vi "Update Numeric Value.vi"(7 "Init Refs":T3, 9 "Tree Data in":cluster{"Tag":string[], "Settings":T1[]} {"Settings"."Data Type" items=["Tree Parent"=-1, "Numeric"=0, "String"=1, "Boolean"=2, "Enum"=3]}, 10 "Settings In":T4, 11 "Tree Tag":string) -> (1 "Tree Data out":cluster{"Tag":string[], "Settings":T1[]} {"Settings"."Data Type" items=["Tree Parent"=-1, "Numeric"=0, "String"=1, "Boolean"=2, "Enum"=3]}, 2 "Settings In out":T4, 3 "New Tree Value":string)   [LabVIEW 2024, in "Sequencer with Output Values.lvlib" / "Sequencer with Output Values.lvclass"]
uses:
  Sequencer with Output Values.lvclass
  Params.ctl
  Step Settings.ctl
  Control Refs.ctl
  Tree Item Settings.ctl
  Data Type.ctl
  Global Tree Data.vi
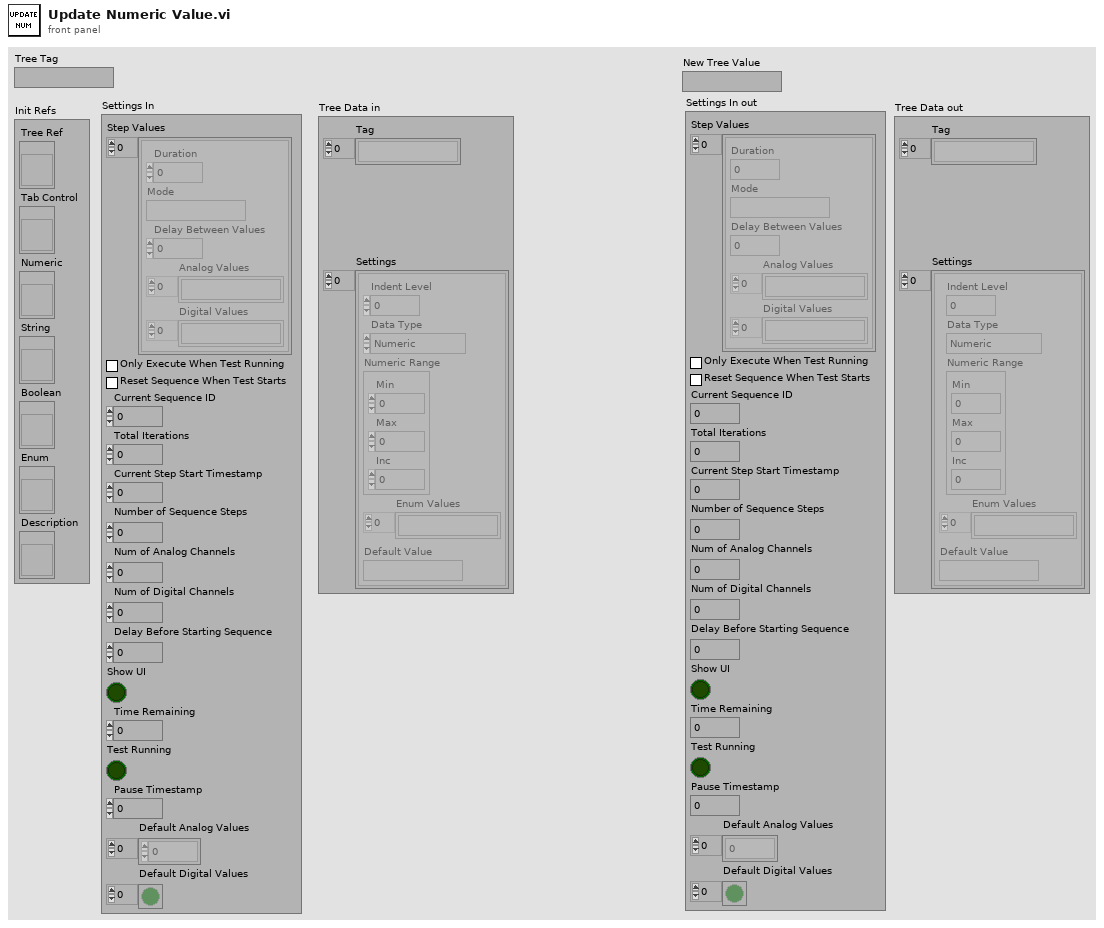
[diagram p1: front panel]
types:
  T1 = typedef "Sequencer with Output Values.lvlib/Sequencer with Output Values.lvclass/Tree Item Settings.ctl" = cluster{"Indent Level":i32, "Data Type":T2, "Numeric Range":cluster{"Min":dbl, "Max":dbl, "Inc":dbl}, "Enum Values":string[], "Default Value":string}
  T2 = typedef "Sequencer with Output Values.lvlib/Sequencer with Output Values.lvclass/Data Type.ctl" = i16
  T3 = typedef "Sequencer with Output Values.lvlib/Sequencer with Output Values.lvclass/Control Refs.ctl" = cluster{"Tree Ref":refnum<vi>, "Tab Control":refnum<vi>, "Numeric":refnum<vi>, "String":refnum<vi>, "Boolean":refnum<vi>, "Enum":refnum<vi>, "Description":refnum<vi>}
  T4 = typedef "Sequencer with Output Values.lvlib/Sequencer with Output Values.lvclass/Params.ctl" = cluster{"Step Values":T5[], "Only Execute When Test Running":bool, "Reset Sequence When Test Starts":bool, "Current Sequence ID":u32, "Total Iterations":u32, "Current Step Start Timestamp":dbl, "Number of Sequence Steps":i32, "Num of Analog Channels":i32, "Num of Digital Channels":i32, "Delay Before Starting Sequence":dbl, "Show UI":bool, "Time Remaining":dbl, "Test Running":bool, "Pause Timestamp":dbl, "Default Analog Values":dbl[], "Default Digital Values":bool[]}
  T5 = typedef "Sequencer with Output Values.lvlib/Sequencer with Output Values.lvclass/Step Settings.ctl" = cluster{"Duration":dbl, "Mode":string, "Delay Between Values":dbl, "Analog Values":string[], "Digital Values":string[]}
  T6 = cluster{"Left Cell String":string, "Child Text":string[], "Child Tag":string, "Item Indent":i32, "Child Only?":bool, "Glyph Index":i32}[]
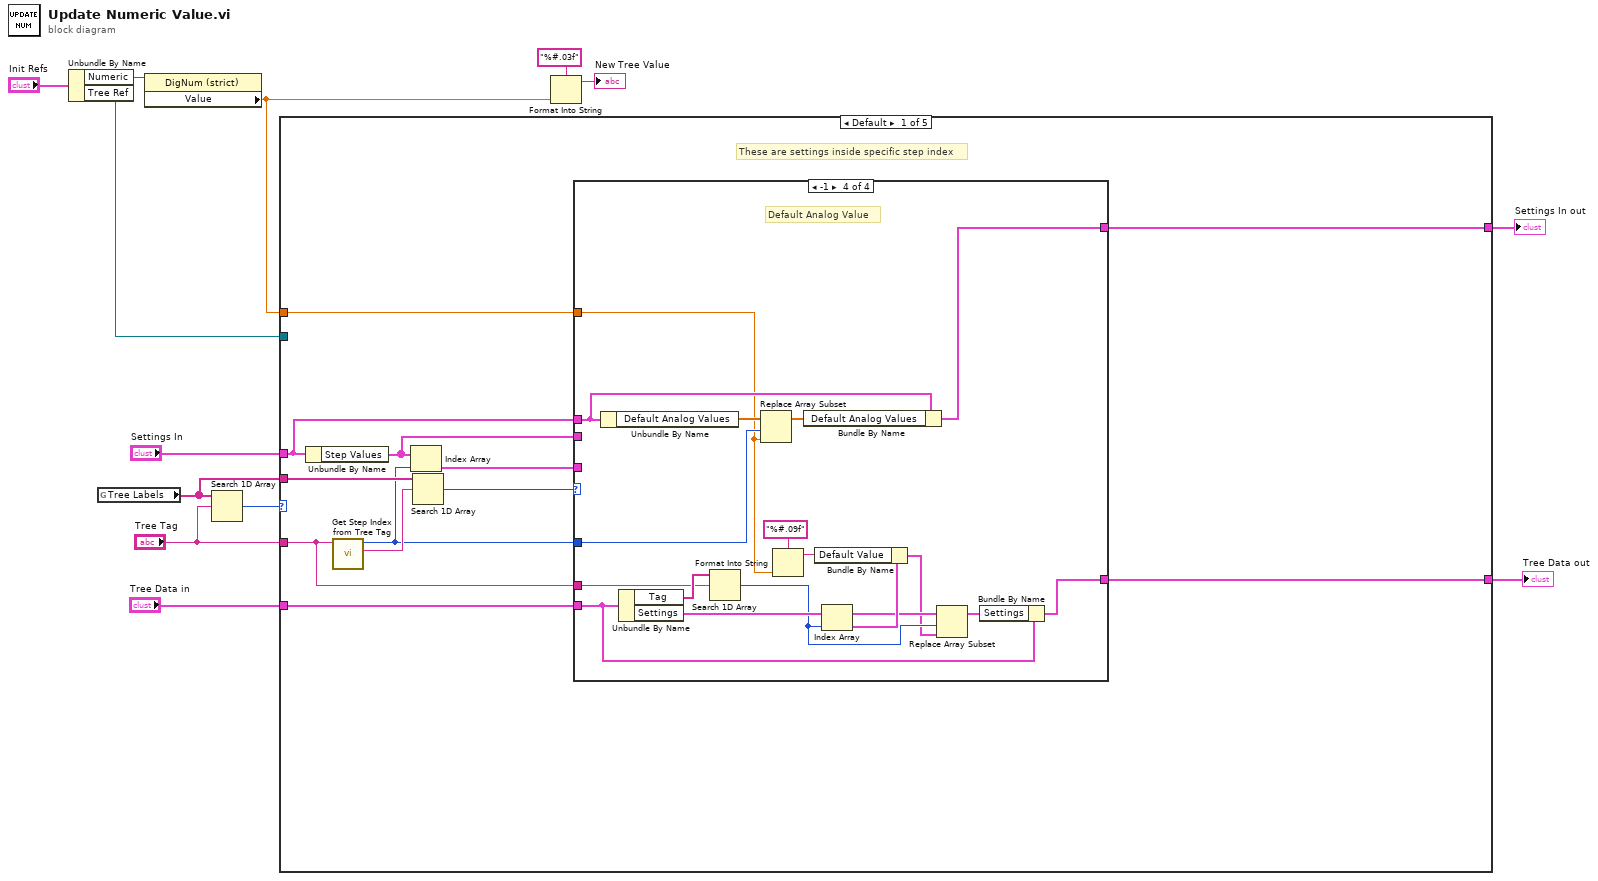
[diagram p0: block diagram]
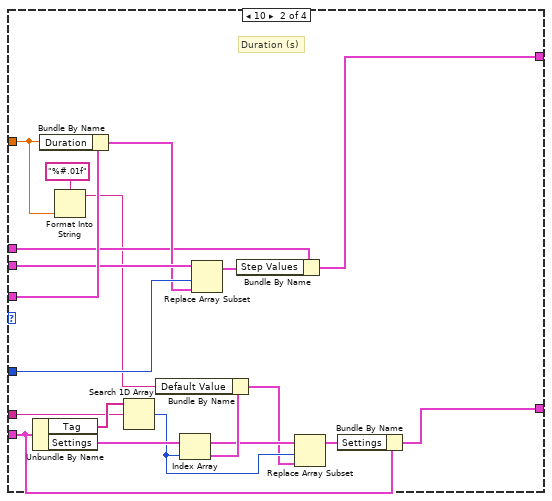
[diagram p3: hidden frame]
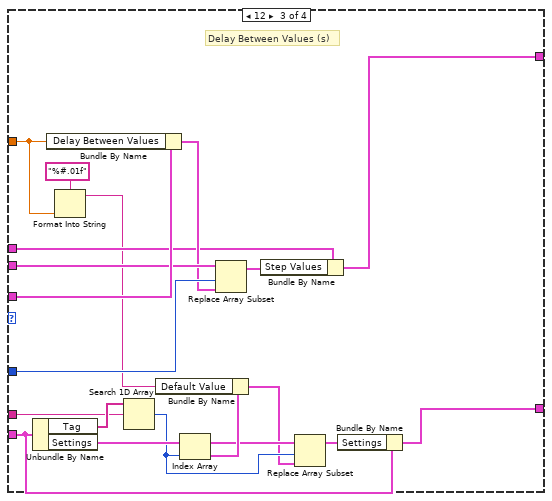
[diagram p4: hidden frame]
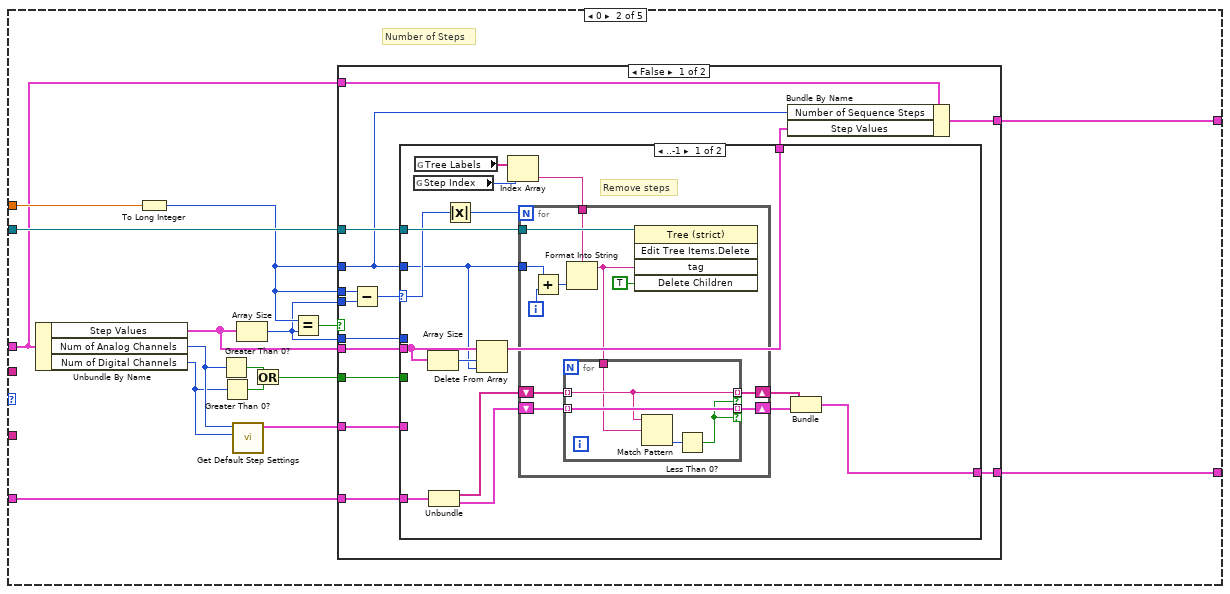
[diagram p5: hidden frame]
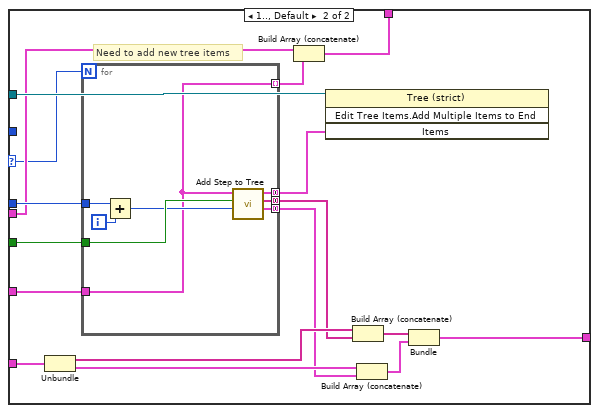
[diagram p6: hidden frame]
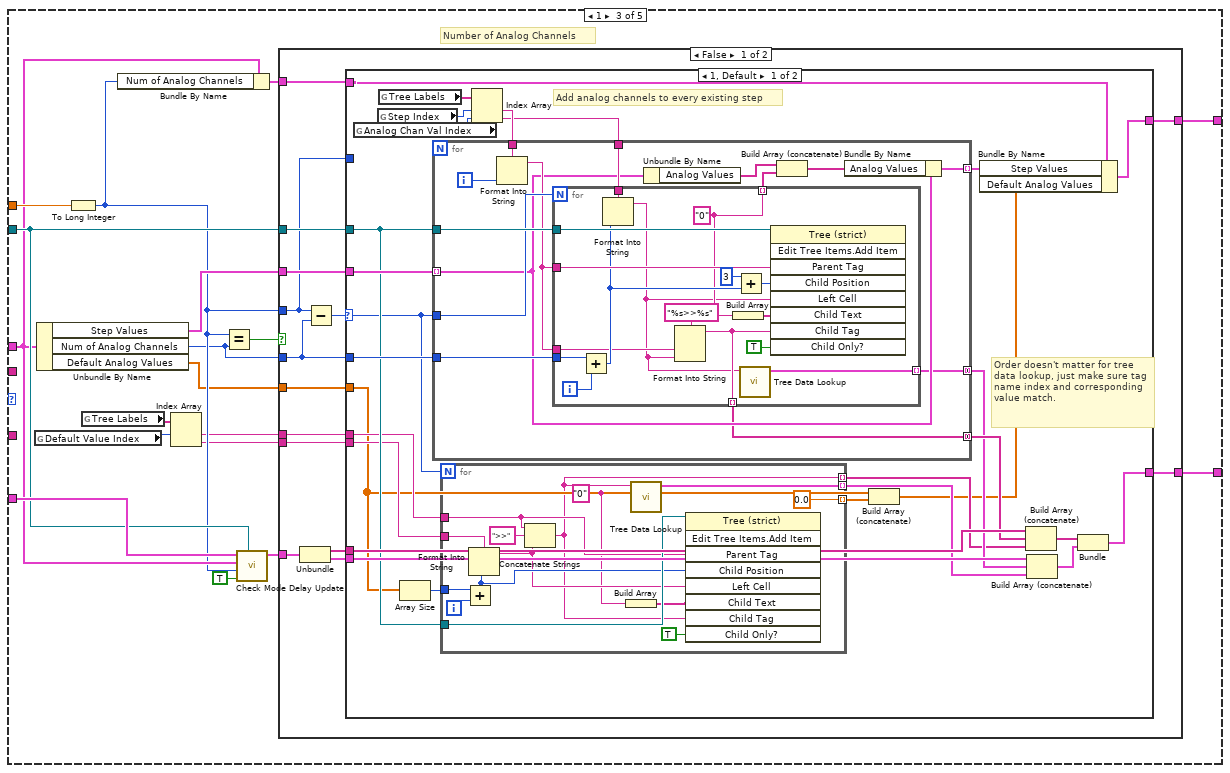
[diagram p8: hidden frame]
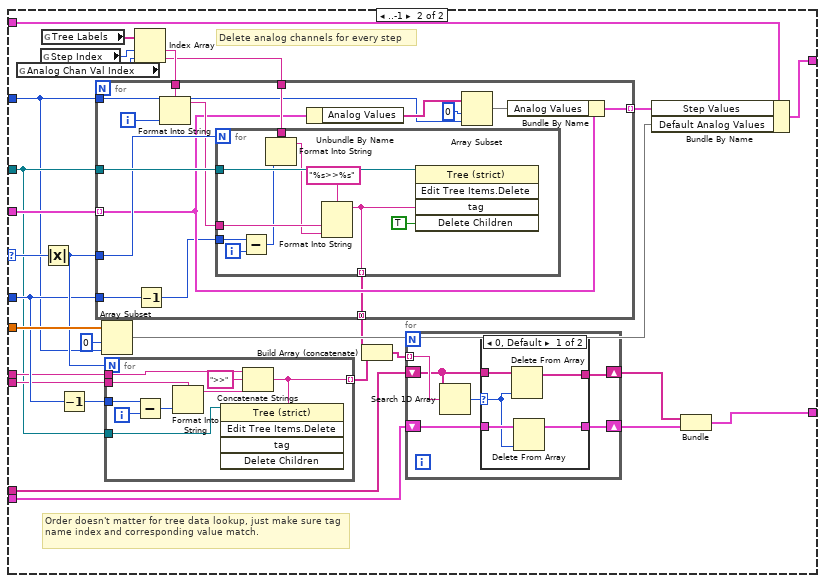
[diagram p9: hidden frame]
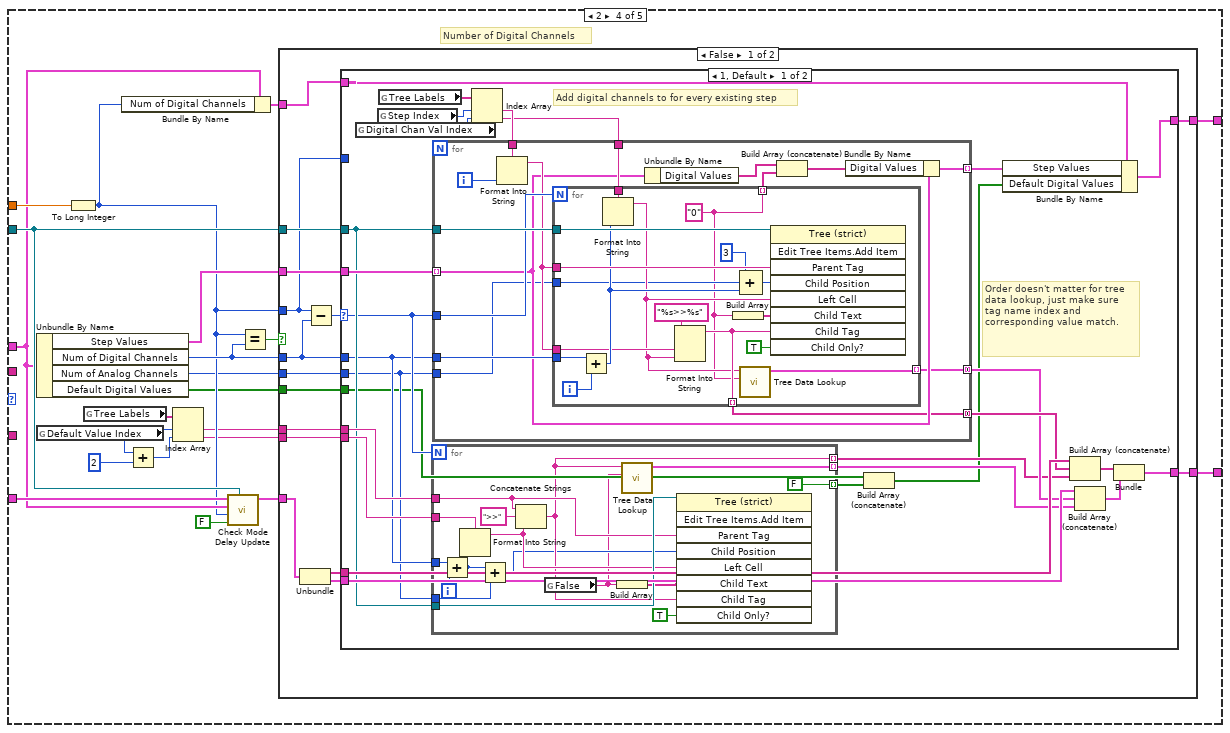
[diagram p12: hidden frame]
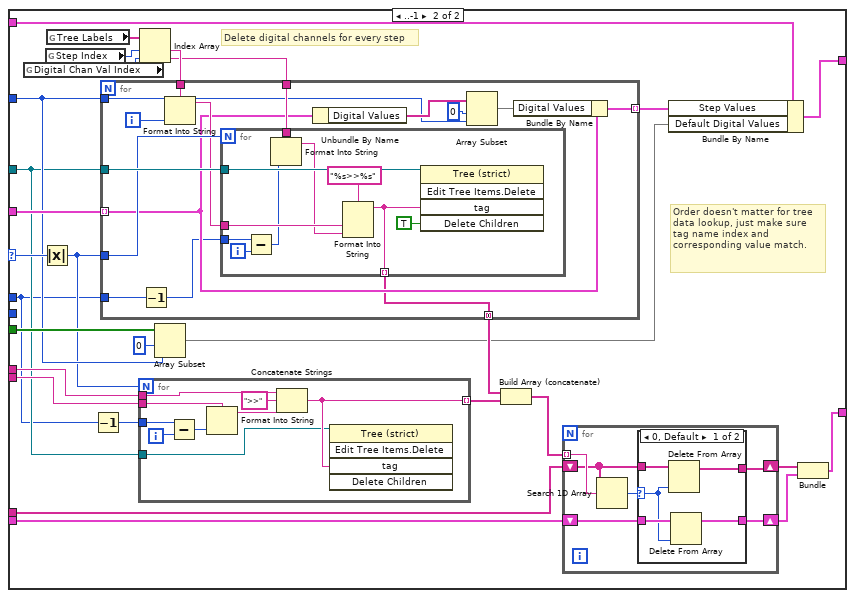
[diagram p13: hidden frame]
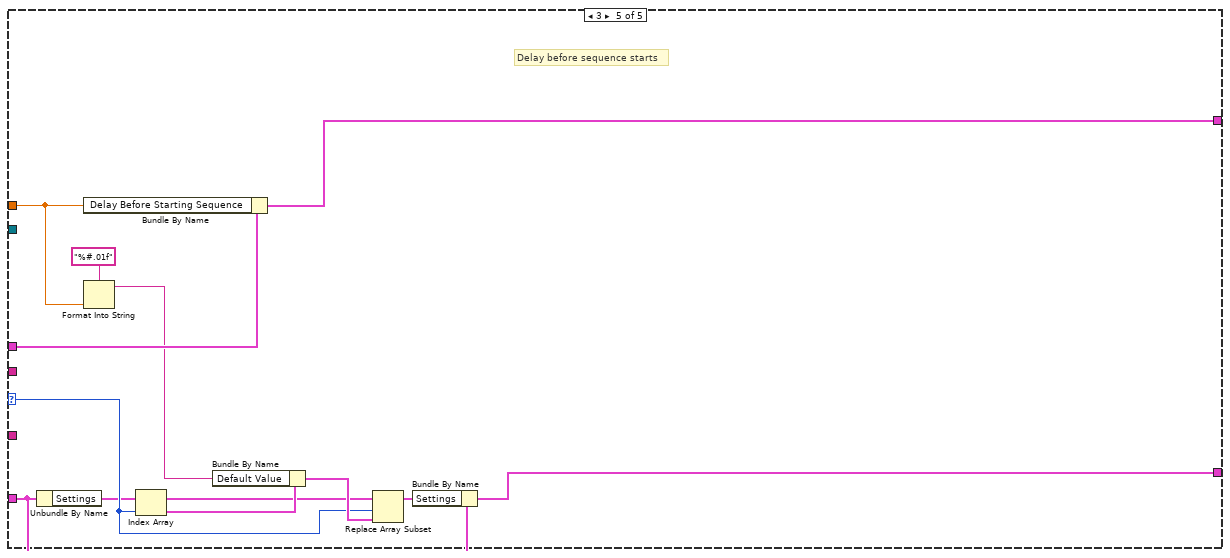
[diagram p16: hidden frame]
diagram:
  n1 = Unbundle By Name("Init Refs") -> ("Numeric"=w11:refnum<vi>, "Tree Ref"=w3:refnum<vi>)
  n2 = global read "Global Tree Data.vi" "Tree Labels"() -> (w1:string[])
  n3 = property class="DigNum (strict)"(reference=w11) -> ("Value"=w8:dbl)  [unwired: 1 in, 2 out]
  n4 = Search 1D Array(1D array=w1, element="Tree Tag") -> (index of element=w9:i32)  [unwired: 1 in]
  n5 = case shown="Default" w9 {
    selector: w9 -> [_ _ _ _ w544]
    tunnel: w8 -> [w21 w98 w189 w372 w548]
    tunnel: w3 -> [_ w96 w182 w363 _]
    tunnel: "Settings In" -> [w19 w87 w180 w362 w551]
    tunnel: "Tree Data in" -> [w20 w89 w183 w365 w543]
    tunnel: [w14 w88 w186 w369 w540] -> w5
    tunnel: [w16 w83 w187 w370 w550] -> w4
    tunnel: "Tree Tag" -> [w15 _ _ _ _]
    tunnel: w1 -> [w25 _ _ _ _]
    frame Default {
      # "These are settings inside specific step index"
      n6 = Unbundle By Name(w19) -> ("Step Values"=w18:T5[])
      n7 = call "Get Step Index from Tree Tag.vi"("Tree Tag"=w15) -> ("Step Param String"=w24:string, "Step Index"=w17:i32)  [unwired: 9 in]
      n8 = Index Array(array=w18, index=w17) -> (element=w23:T5)
      n9 = Search 1D Array(1D array=w25, element=w24) -> (index of element=w22:i32)  [unwired: 1 in]
      n10 = case shown="-1" w22 {
        tunnel: w23 -> [_ w46 w65 _]
        tunnel: w21 -> [_ w36 w55 w68]
        tunnel: w20 -> [w26 w30 w49 w69]
        tunnel: w19 -> [w27 w42 w61 w80]
        tunnel: w18 -> [_ w45 w64 _]
        tunnel: w17 -> [_ w44 w63 w81]
        tunnel: [w27 w40 w59 w78] -> w16
        tunnel: w15 -> [_ w38 w57 w71]
        tunnel: [w26 w28 w47 w70] -> w14
        frame Default {
        }
        frame 10 {
          # "Duration (s)"
          n11 = Unbundle By Name(w30) -> ("Tag"=w39:string[], "Settings"=w33:T1[])
          n12 = Bundle By Name(cluster=w46, "Duration"=w36) -> (w43:T5)
          n13 = Format Into String(format string="%#.01f", w36) -> (resulting string=w34:string)  [unwired: 2 in, 1 out]
          n14 = Search 1D Array(1D array=w39, element=w38) -> (index of element=w32:i32)  [unwired: 1 in]
          n15 = Index Array(array=w33, index=w32) -> (element=w37:T1)
          n16 = Bundle By Name(cluster=w37, "Default Value"=w34) -> (w31:T1)
          n17 = Replace Array Subset(array=w45, new element=w43, index=w44) -> (w41:T5[])
          n18 = Bundle By Name(cluster=w42, "Step Values"=w41) -> (w40:T4)
          n19 = Replace Array Subset(array=w33, new element=w31, index=w32) -> (w29:T1[])
          n20 = Bundle By Name(cluster=w30, "Settings"=w29) -> (w28:cluster{"Tag":string[], "Settings":T1[]})
        }
        frame 12 {
          # "Delay Between Values (s)"
          n21 = Unbundle By Name(w49) -> ("Tag"=w58:string[], "Settings"=w52:T1[])
          n22 = Bundle By Name(cluster=w65, "Delay Between Values"=w55) -> (w62:T5)
          n23 = Format Into String(format string="%#.01f", w55) -> (resulting string=w53:string)  [unwired: 2 in, 1 out]
          n24 = Search 1D Array(1D array=w58, element=w57) -> (index of element=w51:i32)  [unwired: 1 in]
          n25 = Index Array(array=w52, index=w51) -> (element=w56:T1)
          n26 = Bundle By Name(cluster=w56, "Default Value"=w53) -> (w50:T1)
          n27 = Replace Array Subset(array=w64, new element=w62, index=w63) -> (w60:T5[])
          n28 = Bundle By Name(cluster=w61, "Step Values"=w60) -> (w59:T4)
          n29 = Replace Array Subset(array=w52, new element=w50, index=w51) -> (w48:T1[])
          n30 = Bundle By Name(cluster=w49, "Settings"=w48) -> (w47:cluster{"Tag":string[], "Settings":T1[]})
        }
        frame -1 {
          # "Default Analog Value"
          n31 = Unbundle By Name(w80) -> ("Default Analog Values"=w82:dbl[])
          n32 = Unbundle By Name(w69) -> ("Tag"=w77:string[], "Settings"=w75:T1[])
          n33 = Search 1D Array(1D array=w77, element=w71) -> (index of element=w74:i32)  [unwired: 1 in]
          n34 = Replace Array Subset(array=w82, new element=w68, index=w81) -> (w79:dbl[])
          n35 = Format Into String(format string="%#.09f", w68) -> (resulting string=w66:string)  [unwired: 2 in, 1 out]
          n36 = Bundle By Name(cluster=w80, "Default Analog Values"=w79) -> (w78:T4)
          n37 = Index Array(array=w75, index=w74) -> (element=w76:T1)
          n38 = Bundle By Name(cluster=w76, "Default Value"=w66) -> (w73:T1)
          n39 = Replace Array Subset(array=w75, new element=w73, index=w74) -> (w72:T1[])
          n40 = Bundle By Name(cluster=w69, "Settings"=w72) -> (w70:cluster{"Tag":string[], "Settings":T1[]})
        }
      }
    }
    frame 0 {
      # "Number of Steps"
      n41 = Unbundle By Name(w87) -> ("Step Values"=w95:T5[], "Num of Analog Channels"=w86:i32, "Num of Digital Channels"=w85:i32)
      n42 = To Long Integer(number=w98) -> (32bit integer=w94:i32)
      n43 = Greater Than 0?(x=w86) -> (x > 0?=w92:bool)
      n44 = Greater Than 0?(x=w85) -> (x > 0?=w91:bool)
      n45 = call "Get Default Step Settings.vi"("Num of Digital Channels"=w85, "Num of Analog Channels"=w86) -> ("Default Step Settings"=w84:T5)  [unwired: 9 in]
      n46 = Array Size(array=w95) -> (size(s)=w93:i32)
      n47 = Or(x=w92, y=w91) -> (x .or. y?=w90:bool)
      n48 = Equal?(x=w94, y=w93) -> (x = y?=w97:bool)
      n49 = case shown="False" w97 {
        tunnel: w93 -> [w111 _]
        tunnel: w94 -> [w112 _]
        tunnel: w96 -> [w109 _]
        tunnel: w95 -> [w108 _]
        tunnel: w94 -> [w102 _]
        tunnel: w93 -> [w107 _]
        tunnel: w90 -> [w106 _]
        tunnel: w89 -> [w105 w170]
        tunnel: [w104 w170] -> w88
        tunnel: w87 -> [w103 w171]
        tunnel: w84 -> [w101 _]
        tunnel: [w99 w171] -> w83
        frame False {
          n50 = Subtract(x=w112, y=w111) -> (x-y=w110:i32)
          n51 = case shown="..-1" w110 {
            selector: w110 -> [w124 w145]
            tunnel: w109 -> [w125 w159]
            tunnel: w108 -> [w127 w146]
            tunnel: w102 -> [w121 _]
            tunnel: w107 -> [_ w161]
            tunnel: w106 -> [_ w160]
            tunnel: w105 -> [w122 w157]
            tunnel: [w113 w150] -> w104
            tunnel: w101 -> [_ w149]
            tunnel: [w128 w147] -> w100
            frame ..-1 {
              # "Remove steps"
              n52 = global read "Global Tree Data.vi" "Step Index"() -> (w119:i32)
              n53 = global read "Global Tree Data.vi" "Tree Labels"() -> (w120:string[])
              n54 = Array Size(array=w127) -> (size(s)=w126:i32)
              n55 = Unbundle(w122) -> ("Tag"=w117:string[], "Settings"=w116:T1[])
              n56 = Absolute Value(x=w124) -> (abs(x)=w123:i32)
              n57 = Delete From Array(array=w127, length=w126, index=w121) -> (array with subset deleted=w128:T5[])  [unwired: 1 out]
              n58 = Index Array(array=w120, index=w119) -> (element=w118:string)
              n59 = for {
                N: w123 -> [_]
                tunnel: w125 -> [w139]
                tunnel: w121 -> [w137]
                tunnel: w118 -> [w134]
                shift-right: [w131] -> w115
                shift-left: w117 -> [w133]
                shift-right: [w130] -> w114
                shift-left: w116 -> [w132]
                i -> [w136]
                n60 = Add(x=w137, y=w136) -> (x+y=w135:i32)
                n61 = Format Into String(format string=w134, w135) -> (resulting string=w129:string)  [unwired: 2 in, 1 out]
                n62 = for {
                  tunnel: w133 -> [w143] mode=indexing
                  tunnel: w132 -> [w144] mode=indexing
                  tunnel: [w143] -> w131 mode=indexing if=w140
                  tunnel: [w144] -> w130 mode=indexing if=w140
                  tunnel: w129 -> [w142]
                  n63 = Match Pattern(string=w143, regular expression=w142) -> (offset past match=w141:i32)  [unwired: 1 in, 3 out]
                  n64 = Less Than 0?(x=w141) -> (x < 0?=w140:bool)
                }
                n65 = invoke class="Tree (strict)" method="Edit Tree Items.Delete"(reference=w139, "tag"=w129, "Delete Children"=TRUE ("Delete Children?")) -> ()  [unwired: 2 in, 5 out]
              }
              n66 = Bundle("Tag"=w115, "Settings"=w114) -> (w113:cluster{"Tag":string[], "Settings":T1[]})  [unwired: 1 in]
            }
            frame 1.., Default {
              # "Need to add new tree items"
              n67 = Unbundle(w157) -> ("Tag"=w156:string[], "Settings"=w154:T1[])
              n68 = for {
                N: w145 -> [_]
                tunnel: w161 -> [w169]
                tunnel: w160 -> [w167]
                tunnel: [w165] -> w158 mode=concatenating
                tunnel: [w164] -> w155 mode=concatenating
                tunnel: [w163] -> w153 mode=concatenating
                tunnel: w149 -> [w162]
                tunnel: [w162] -> w148 mode=indexing
                i -> [w168]
                n69 = Add(x=w169, y=w168) -> (x+y=w166:i32)
                n70 = call "Add Step to Tree.vi"("Step Index"=w166, "Channels Defined"=w167, "Step Settings"=w162) -> ("Tree Data"=w163:T1[], "Tree Tags"=w164:string[], "Tree Items"=w165:T6)  [unwired: 6 in]
              }
              n71 = Build Array (concatenate)(w146, w148) -> (w147:T5[])
              n72 = invoke class="Tree (strict)" method="Edit Tree Items.Add Multiple Items to End"(reference=w159, "Items"=w158) -> ()  [unwired: 2 in, 4 out]
              n73 = Build Array (concatenate)(w156, w155) -> (w152:string[])
              n74 = Build Array (concatenate)(w154, w153) -> (w151:T1[])
              n75 = Bundle(w152, w151) -> (w150:cluster{string[], T1[]})  [unwired: 1 in]
            }
          }
          n76 = Bundle By Name(cluster=w103, "Number of Sequence Steps"=w102, "Step Values"=w100) -> (w99:T4)
        }
        frame True {
          # "Didn't change, so nothing to do."
        }
      }
    }
    frame 1 {
      # "Number of Analog Channels"
      n77 = global read "Global Tree Data.vi" "Default Value Index"() -> (w174:i32)
      n78 = Unbundle By Name(w180) -> ("Step Values"=w185:T5[], "Num of Analog Channels"=w177:i32, "Default Analog Values"=w176:dbl[])
      n79 = To Long Integer(number=w189) -> (32bit integer=w179:i32)
      n80 = global read "Global Tree Data.vi" "Tree Labels"() -> (w175:string[])
      n81 = Bundle By Name(cluster=w180, "Num of Analog Channels"=w179) -> (w178:T4)
      n82 = Index Array(array=w175, index #1=w174) -> (element #1=w172:string, element #2=w173:string)  [unwired: 1 in]
      n83 = Equal?(x=w179, y=w177) -> (x = y?=w188:bool)
      n84 = call "Check Mode Delay Update.vi"("TreeControl in"=w182, "Analog Changed"=TRUE, "New Num"=w179, "Settings In in"=w180, "Tree Data in"=w183) -> ("Tree Data out"=w184:cluster{"Tag":string[], "Settings":T1[]})  [unwired: 6 in]
      n85 = case shown="False" w188 {
        tunnel: w178 -> [w199 w351]
        tunnel: [w198 w351] -> w187
        tunnel: w184 -> [w197 w350]
        tunnel: [w194 w350] -> w186
        tunnel: w177 -> [w200 _]
        tunnel: w179 -> [w193 _]
        tunnel: w182 -> [w202 _]
        tunnel: w185 -> [w201 _]
        tunnel: w176 -> [w192 _]
        tunnel: w173 -> [w191 _]
        tunnel: w172 -> [w190 _]
        frame False {
          n86 = Unbundle(w197) -> ("Tag"=w196:string[], "Settings"=w195:T1[])
          n87 = Subtract(x=w193, y=w200) -> (x-y=w203:i32)
          n88 = case shown="1, Default" w203 {
            selector: w203 -> [w208 w298]
            tunnel: w202 -> [w211 w276]
            tunnel: w201 -> [w230 w302]
            tunnel: w200 -> [w226 w281]
            tunnel: w199 -> [w223 w295]
            tunnel: [w221 w293] -> w198
            tunnel: w196 -> [w220 w291]
            tunnel: w195 -> [w218 w290]
            tunnel: [w214 w292] -> w194
            tunnel: w193 -> [_ w275]
            tunnel: w192 -> [w205 w287]
            tunnel: w191 -> [w209 w279]
            tunnel: w190 -> [w210 w277]
            frame 1, Default {
              # "Order doesn't matter for tree data lookup, just make sure tag name index and corresponding value match."
              # "Add analog channels to every existing step"
              n89 = global read "Global Tree Data.vi" "Analog Chan Val Index"() -> (w225:i32)
              n90 = global read "Global Tree Data.vi" "Step Index"() -> (w229:i32)
              n91 = global read "Global Tree Data.vi" "Tree Labels"() -> (w228:string[])
              n92 = Array Size(array=w205) -> (size(s)=w207:i32)
              n93 = for {
                N: w208 -> [_]
                tunnel: [w243] -> w212 mode=indexing
                tunnel: [w233] -> w213 mode=indexing
                tunnel: w211 -> [w242]
                tunnel: w210 -> [w238]
                tunnel: w209 -> [w241]
                tunnel: w207 -> [w239]
                tunnel: [0.0] -> w206 mode=indexing
                i -> [w240]
                w235 = "0" ("Value")
                n94 = Add(x=w239, y=w240) -> (x+y=w237:i32)
                n95 = Format Into String(format string=w241, w237) -> (resulting string=w236:string)  [unwired: 2 in, 1 out]
                n96 = Concatenate Strings(w238, ">>" ("string"), w236) -> (w233:string)
                n97 = Build Array(w235) -> (w234:string[])
                n98 = call "Tree Data Lookup.vi"("Value"=w235, "Key"=w233) -> ("Tree Data"=w243:T1)  [unwired: 9 in]
                n99 = invoke class="Tree (strict)" method="Edit Tree Items.Add Item"(reference=w242, "Parent Tag"=w238, "Child Position"=w237, "Left Cell"=w236, "Child Text"=w234, "Child Tag"=w233, "Child Only?"=TRUE) -> ()  [unwired: 2 in, 9 out]
              }
              n100 = Index Array(array=w228, index #1=w229, index #2=w225) -> (element #1=w227:string, element #2=w224:string)
              n101 = for {
                tunnel: w211 -> [w258]
                tunnel: w230 -> [w251] mode=indexing
                tunnel: w227 -> [w257]
                tunnel: w226 -> [w255]
                tunnel: w208 -> [w254]
                tunnel: w224 -> [w253]
                tunnel: [w247] -> w222 mode=indexing
                tunnel: [w246] -> w219 mode=concatenating
                tunnel: [w245] -> w217 mode=concatenating
                i -> [w256]
                n102 = Format Into String(format string=w257, w256) -> (resulting string=w252:string)  [unwired: 2 in, 1 out]
                n103 = for {
                  N: w254 -> [_]
                  tunnel: w258 -> [w274]
                  tunnel: w255 -> [w273]
                  tunnel: w253 -> [w271]
                  tunnel: w252 -> [w270]
                  tunnel: w252 -> [w265]
                  tunnel: [w263] -> w249 mode=indexing
                  tunnel: [w262] -> w246 mode=indexing
                  tunnel: [w260] -> w245 mode=indexing
                  i -> [w272]
                  w263 = "0"
                  n104 = Add(x=w273, y=w272) -> (x+y=w268:i32)
                  n105 = Format Into String(format string=w271, w268) -> (resulting string=w261:string)  [unwired: 2 in, 1 out]
                  n106 = Format Into String(format string="%s>>%s" ("string"), w265, w261) -> (resulting string=w262:string)  [unwired: 2 in, 1 out]
                  n107 = Build Array(w263) -> (w259:string[])
                  n108 = Add(x=3, y=w268) -> (x+y=w267:i32)
                  n109 = call "Tree Data Lookup.vi"("Key"=w261) -> ("Tree Data"=w260:T1)  [unwired: 10 in]
                  n110 = invoke class="Tree (strict)" method="Edit Tree Items.Add Item"(reference=w274, "Parent Tag"=w270, "Child Position"=w267, "Left Cell"=w261, "Child Text"=w259, "Child Tag"=w262, "Child Only?"=TRUE) -> ()  [unwired: 2 in, 9 out]
                }
                n111 = Unbundle By Name(w251) -> ("Analog Values"=w250:string[])
                n112 = Build Array (concatenate)(w250, w249) -> (w248:string[])
                n113 = Bundle By Name(cluster=w251, "Analog Values"=w248) -> (w247:T5)
              }
              n114 = Build Array (concatenate)(w205, w206) -> (w204:dbl[])
              n115 = Bundle By Name(cluster=w223, "Step Values"=w222, "Default Analog Values"=w204) -> (w221:T4)
              n116 = Build Array (concatenate)(w220, w219, w213) -> (w216:string[])
              n117 = Build Array (concatenate)(w218, w217, w212) -> (w215:T1[])
              n118 = Bundle(w216, w215) -> (w214:cluster{string[], T1[]})  [unwired: 1 in]
            }
            frame ..-1 {
              # "Order doesn't matter for tree data lookup, just make sure tag name index and corresponding value match."
              # "Delete analog channels for every step"
              n119 = global read "Global Tree Data.vi" "Analog Chan Val Index"() -> (w297:i32)
              n120 = global read "Global Tree Data.vi" "Step Index"() -> (w301:i32)
              n121 = global read "Global Tree Data.vi" "Tree Labels"() -> (w300:string[])
              n122 = Absolute Value(x=w298) -> (abs(x)=w284:i32)
              n123 = Decrement(x=w281) -> (x-1=w280:i32)
              n124 = Array Subset(array=w287, index=0, length=w275) -> (w285:dbl[])
              n125 = for {
                N: w284 -> [_]
                tunnel: w280 -> [w311]
                tunnel: w279 -> [w308]
                tunnel: w277 -> [w306]
                tunnel: [w304] -> w278 mode=indexing
                tunnel: w276 -> [w303]
                i -> [w310]
                n126 = Subtract(x=w311, y=w310) -> (x-y=w309:i32)
                n127 = Format Into String(format string=w308, w309) -> (resulting string=w305:string)  [unwired: 2 in, 1 out]
                n128 = Concatenate Strings(w306, ">>" ("string"), w305) -> (w304:string)
                n129 = invoke class="Tree (strict)" method="Edit Tree Items.Delete"(reference=w303, "tag"=w304) -> ()  [unwired: 3 in, 5 out]
              }
              n130 = Index Array(array=w300, index #1=w301, index #2=w297) -> (element #1=w299:string, element #2=w296:string)
              n131 = for {
                tunnel: w276 -> [w339]
                tunnel: w302 -> [w332] mode=indexing
                tunnel: w299 -> [w338]
                tunnel: w281 -> [w336]
                tunnel: w284 -> [w335]
                tunnel: w296 -> [w334]
                tunnel: [w331] -> w294 mode=indexing
                tunnel: [w330] -> w283 mode=concatenating
                tunnel: w275 -> [w326]
                i -> [w337]
                n132 = Decrement(x=w336) -> (x-1=w329:i32)
                n133 = Format Into String(format string=w338, w337) -> (resulting string=w333:string)  [unwired: 2 in, 1 out]
                n134 = for {
                  N: w335 -> [_]
                  tunnel: w339 -> [w349]
                  tunnel: w329 -> [w345]
                  tunnel: w334 -> [w348]
                  tunnel: w333 -> [w347]
                  tunnel: [w341] -> w330 mode=indexing
                  i -> [w344]
                  n135 = Subtract(x=w345, y=w344) -> (x-y=w343:i32)
                  n136 = Format Into String(format string=w348, w343) -> (resulting string=w346:string)  [unwired: 2 in, 1 out]
                  n137 = Format Into String(format string="%s>>%s", w347, w346) -> (resulting string=w341:string)  [unwired: 2 in, 1 out]
                  n138 = invoke class="Tree (strict)" method="Edit Tree Items.Delete"(reference=w349, "tag"=w341, "Delete Children"=TRUE ("Delete Children?")) -> ()  [unwired: 2 in, 5 out]
                }
                n139 = Unbundle By Name(w332) -> ("Analog Values"=w328:string[])
                n140 = Array Subset(array=w328, index=0, length=w326) -> (w327:string[])
                n141 = Bundle By Name(cluster=w332, "Analog Values"=w327) -> (w331:T5)
              }
              n142 = Build Array (concatenate)(w283, w278) -> (w282:string[])
              n143 = for {
                tunnel: w282 -> [w317] mode=indexing
                shift-right: [w314] -> w289
                shift-left: w291 -> [w315]
                shift-right: [w312] -> w288
                shift-left: w290 -> [w313]
                n144 = Search 1D Array(1D array=w315, element=w317) -> (index of element=w316:i32)  [unwired: 1 in]
                n145 = case shown="0, Default" w316 {
                  selector: w316 -> [w319 _]
                  tunnel: w315 -> [w322 w324]
                  tunnel: [w321 w324] -> w314
                  tunnel: w313 -> [w320 w323]
                  tunnel: [w318 w323] -> w312
                  frame 0, Default {
                    n146 = Delete From Array(array=w322, index=w319) -> (array with subset deleted=w321:string[])  [unwired: 1 in, 1 out]
                    n147 = Delete From Array(array=w320, index=w319) -> (array with subset deleted=w318:T1[])  [unwired: 1 in, 1 out]
                  }
                  frame -1 {
                  }
                }
              }
              n148 = Bundle By Name(cluster=w295, "Step Values"=w294, "Default Analog Values"=w285) -> (w293:T4)
              n149 = Bundle("Tag"=w289, "Settings"=w288) -> (w292:cluster{"Tag":string[], "Settings":T1[]})  [unwired: 1 in]
            }
          }
        }
        frame True {
        }
      }
    }
    frame 2 {
      # "Number of Digital Channels"
      n150 = Unbundle By Name(w362) -> ("Step Values"=w368:T5[], "Num of Digital Channels"=w367:i32, "Num of Analog Channels"=w359:i32, "Default Digital Values"=w352:bool[])
      n151 = global read "Global Tree Data.vi" "Default Value Index"() -> (w357:i32)
      n152 = To Long Integer(number=w372) -> (32bit integer=w361:i32)
      n153 = global read "Global Tree Data.vi" "Tree Labels"() -> (w358:string[])
      n154 = Bundle By Name(cluster=w362, "Num of Digital Channels"=w361) -> (w360:T4)
      n155 = Add(x=w357, y=2) -> (x+y=w355:i32)
      n156 = Index Array(array=w358, index #1=w357, index #2=w355) -> (element #1=w354:string, element #2=w353:string)
      n157 = call "Check Mode Delay Update.vi"("TreeControl in"=w363, "Analog Changed"=FALSE, "New Num"=w361, "Settings In in"=w362, "Tree Data in"=w365) -> ("Tree Data out"=w364:cluster{"Tag":string[], "Settings":T1[]})  [unwired: 6 in]
      n158 = Equal?(x=w361, y=w367) -> (x = y?=w371:bool)
      n159 = case shown="False" w371 {
        tunnel: w360 -> [w383 w539]
        tunnel: [w382 w539] -> w370
        tunnel: w364 -> [w381 w538]
        tunnel: [w378 w538] -> w369
        tunnel: w367 -> [w384 _]
        tunnel: w361 -> [w377 _]
        tunnel: w363 -> [w386 _]
        tunnel: w368 -> [w385 _]
        tunnel: w359 -> [w376 _]
        tunnel: w354 -> [w375 _]
        tunnel: w353 -> [w374 _]
        tunnel: w352 -> [w373 _]
        frame False {
          n160 = Unbundle(w381) -> ("Tag"=w380:string[], "Settings"=w379:T1[])
          n161 = Subtract(x=w377, y=w384) -> (x-y=w387:i32)
          n162 = case shown="1, Default" w387 {
            selector: w387 -> [w395 w486]
            tunnel: w386 -> [w396 w465]
            tunnel: w385 -> [w414 w490]
            tunnel: w384 -> [w394 w463]
            tunnel: w383 -> [w408 w483]
            tunnel: [w406 w481] -> w382
            tunnel: w380 -> [w405 w479]
            tunnel: w379 -> [w403 w478]
            tunnel: [w399 w480] -> w378
            tunnel: w377 -> [_ w470]
            tunnel: w376 -> [w393 _]
            tunnel: w375 -> [w398 w467]
            tunnel: w374 -> [w397 w466]
            tunnel: w373 -> [w389 w472]
            frame 1, Default {
              # "Order doesn't matter for tree data lookup, just make sure tag name index and corresponding value match."
              # "Add digital channels to for every existing step"
              n163 = global read "Global Tree Data.vi" "Digital Chan Val Index"() -> (w410:i32)
              n164 = global read "Global Tree Data.vi" "Step Index"() -> (w413:i32)
              n165 = global read "Global Tree Data.vi" "Tree Labels"() -> (w412:string[])
              n166 = for {
                N: w395 -> [_]
                tunnel: [w429] -> w391 mode=indexing
                tunnel: [w421] -> w392 mode=indexing
                tunnel: w396 -> [w428]
                tunnel: w398 -> [w424]
                tunnel: w397 -> [w427]
                tunnel: w394 -> [w425]
                tunnel: [FALSE] -> w390 mode=indexing
                tunnel: w393 -> [w417]
                i -> [w426]
                n167 = Add(x=w425, y=w426) -> (x+y=w418:i32)
                n168 = Format Into String(format string=w427, w418) -> (resulting string=w423:string)  [unwired: 2 in, 1 out]
                n169 = Add(x=w418, y=w417) -> (x+y=w416:i32)
                n170 = Concatenate Strings(w424, ">>" ("string"), w423) -> (w421:string)
                n171 = global read "Global Tree Data.vi" "False"() -> (w415:string)
                n172 = Build Array(w415) -> (w422:string[])
                n173 = call "Tree Data Lookup.vi"("Value"=w415, "Key"=w421) -> ("Tree Data"=w429:T1)  [unwired: 9 in]
                n174 = invoke class="Tree (strict)" method="Edit Tree Items.Add Item"(reference=w428, "Parent Tag"=w424, "Child Position"=w416, "Left Cell"=w423, "Child Text"=w422, "Child Tag"=w421, "Child Only?"=TRUE) -> ()  [unwired: 2 in, 9 out]
              }
              n175 = Index Array(array=w412, index #1=w413, index #2=w410) -> (element #1=w411:string, element #2=w409:string)
              n176 = for {
                tunnel: w396 -> [w445]
                tunnel: w414 -> [w438] mode=indexing
                tunnel: w411 -> [w444]
                tunnel: w394 -> [w442]
                tunnel: w395 -> [w441]
                tunnel: w409 -> [w440]
                tunnel: [w434] -> w407 mode=indexing
                tunnel: [w433] -> w404 mode=concatenating
                tunnel: [w432] -> w402 mode=concatenating
                tunnel: w393 -> [w431]
                i -> [w443]
                n177 = Format Into String(format string=w444, w443) -> (resulting string=w439:string)  [unwired: 2 in, 1 out]
                n178 = for {
                  N: w441 -> [_]
                  tunnel: w445 -> [w462]
                  tunnel: w442 -> [w461]
                  tunnel: w440 -> [w459]
                  tunnel: w439 -> [w458]
                  tunnel: w439 -> [w454]
                  tunnel: [w446] -> w436 mode=indexing
                  tunnel: [w452] -> w433 mode=indexing
                  tunnel: [w450] -> w432 mode=indexing
                  tunnel: w431 -> [w447]
                  i -> [w460]
                  w446 = "0"
                  n179 = Add(x=w461, y=w460) -> (x+y=w457:i32)
                  n180 = Format Into String(format string=w459, w457) -> (resulting string=w451:string)  [unwired: 2 in, 1 out]
                  n181 = Format Into String(format string="%s>>%s" ("string"), w454, w451) -> (resulting string=w452:string)  [unwired: 2 in, 1 out]
                  n182 = Build Array(w446) -> (w449:string[])
                  n183 = Compound Arithmetic op=ADD(3, w447, w457) -> (w456:i32)
                  n184 = call "Tree Data Lookup.vi"("Value"=w446, "Key"=w451) -> ("Tree Data"=w450:T1)  [unwired: 9 in]
                  n185 = invoke class="Tree (strict)" method="Edit Tree Items.Add Item"(reference=w462, "Parent Tag"=w458, "Child Position"=w456, "Left Cell"=w451, "Child Text"=w449, "Child Tag"=w452, "Child Only?"=TRUE) -> ()  [unwired: 2 in, 9 out]
                }
                n186 = Unbundle By Name(w438) -> ("Digital Values"=w437:string[])
                n187 = Build Array (concatenate)(w437, w436) -> (w435:string[])
                n188 = Bundle By Name(cluster=w438, "Digital Values"=w435) -> (w434:T5)
              }
              n189 = Build Array (concatenate)(w389, w390) -> (w388:bool[])
              n190 = Bundle By Name(cluster=w408, "Step Values"=w407, "Default Digital Values"=w388) -> (w406:T4)
              n191 = Build Array (concatenate)(w405, w404, w392) -> (w401:string[])
              n192 = Build Array (concatenate)(w403, w402, w391) -> (w400:T1[])
              n193 = Bundle(w401, w400) -> (w399:cluster{string[], T1[]})  [unwired: 1 in]
            }
            frame ..-1 {
              # "Order doesn't matter for tree data lookup, just make sure tag name index and corresponding value match."
              # "Delete digital channels for every step"
              n194 = global read "Global Tree Data.vi" "Digital Chan Val Index"() -> (w485:i32)
              n195 = Absolute Value(x=w486) -> (abs(x)=w469:i32)
              n196 = global read "Global Tree Data.vi" "Step Index"() -> (w489:i32)
              n197 = global read "Global Tree Data.vi" "Tree Labels"() -> (w488:string[])
              n198 = Decrement(x=w463) -> (x-1=w464:i32)
              n199 = for {
                N: w469 -> [_]
                tunnel: w464 -> [w499]
                tunnel: w466 -> [w496]
                tunnel: w467 -> [w494]
                tunnel: [w492] -> w473 mode=indexing
                tunnel: w465 -> [w491]
                i -> [w498]
                n200 = Subtract(x=w499, y=w498) -> (x-y=w497:i32)
                n201 = Format Into String(format string=w496, w497) -> (resulting string=w493:string)  [unwired: 2 in, 1 out]
                n202 = Concatenate Strings(w494, ">>" ("string"), w493) -> (w492:string)
                n203 = invoke class="Tree (strict)" method="Edit Tree Items.Delete"(reference=w491, "tag"=w492) -> ()  [unwired: 3 in, 5 out]
              }
              n204 = Index Array(array=w488, index #1=w489, index #2=w485) -> (element #1=w487:string, element #2=w484:string)
              n205 = for {
                tunnel: w465 -> [w527]
                tunnel: w490 -> [w520] mode=indexing
                tunnel: w487 -> [w526]
                tunnel: w463 -> [w524]
                tunnel: w469 -> [w523]
                tunnel: w484 -> [w522]
                tunnel: [w519] -> w482 mode=indexing
                tunnel: [w518] -> w475 mode=concatenating
                tunnel: w470 -> [w514]
                i -> [w525]
                n206 = Decrement(x=w524) -> (x-1=w517:i32)
                n207 = Format Into String(format string=w526, w525) -> (resulting string=w521:string)  [unwired: 2 in, 1 out]
                n208 = for {
                  N: w523 -> [_]
                  tunnel: w527 -> [w537]
                  tunnel: w517 -> [w533]
                  tunnel: w522 -> [w536]
                  tunnel: w521 -> [w535]
                  tunnel: [w529] -> w518 mode=indexing
                  i -> [w532]
                  n209 = Subtract(x=w533, y=w532) -> (x-y=w531:i32)
                  n210 = Format Into String(format string=w536, w531) -> (resulting string=w534:string)  [unwired: 2 in, 1 out]
                  n211 = Format Into String(format string="%s>>%s", w535, w534) -> (resulting string=w529:string)  [unwired: 2 in, 1 out]
                  n212 = invoke class="Tree (strict)" method="Edit Tree Items.Delete"(reference=w537, "tag"=w529, "Delete Children"=TRUE ("Delete Children?")) -> ()  [unwired: 2 in, 5 out]
                }
                n213 = Unbundle By Name(w520) -> ("Digital Values"=w516:string[])
                n214 = Array Subset(array=w516, index=0, length=w514) -> (w515:string[])
                n215 = Bundle By Name(cluster=w520, "Digital Values"=w515) -> (w519:T5)
              }
              n216 = Array Subset(array=w472, index=0, length=w470) -> (w468:bool[])
              n217 = Build Array (concatenate)(w475, w473) -> (w474:string[])
              n218 = for {
                tunnel: w474 -> [w505] mode=indexing
                shift-right: [w502] -> w477
                shift-left: w479 -> [w503]
                shift-right: [w500] -> w476
                shift-left: w478 -> [w501]
                n219 = Search 1D Array(1D array=w503, element=w505) -> (index of element=w504:i32)  [unwired: 1 in]
                n220 = case shown="0, Default" w504 {
                  selector: w504 -> [w507 _]
                  tunnel: w503 -> [w510 w512]
                  tunnel: [w509 w512] -> w502
                  tunnel: w501 -> [w508 w511]
                  tunnel: [w506 w511] -> w500
                  frame 0, Default {
                    n221 = Delete From Array(array=w510, index=w507) -> (array with subset deleted=w509:string[])  [unwired: 1 in, 1 out]
                    n222 = Delete From Array(array=w508, index=w507) -> (array with subset deleted=w506:T1[])  [unwired: 1 in, 1 out]
                  }
                  frame -1 {
                  }
                }
              }
              n223 = Bundle By Name(cluster=w483, "Step Values"=w482, "Default Digital Values"=w468) -> (w481:T4)
              n224 = Bundle("Tag"=w477, "Settings"=w476) -> (w480:cluster{"Tag":string[], "Settings":T1[]})  [unwired: 1 in]
            }
          }
        }
        frame True {
        }
      }
    }
    frame 3 {
      # "Delay before sequence starts"
      n225 = Unbundle By Name(w543) -> ("Settings"=w542:T1[])
      n226 = Bundle By Name(cluster=w551, "Delay Before Starting Sequence"=w548) -> (w550:T4)
      n227 = Format Into String(format string="%#.01f", w548) -> (resulting string=w546:string)  [unwired: 2 in, 1 out]
      n228 = Index Array(array=w542, index=w544) -> (element=w549:T1)
      n229 = Bundle By Name(cluster=w549, "Default Value"=w546) -> (w545:T1)
      n230 = Replace Array Subset(array=w542, new element=w545, index=w544) -> (w541:T1[])
      n231 = Bundle By Name(cluster=w543, "Settings"=w541) -> (w540:cluster{"Tag":string[], "Settings":T1[]})
    }
  }
  "Settings In out" <- w4
  "Tree Data out" <- w5
  n232 = Format Into String(format string="%#.03f", w8) -> (resulting string=→"New Tree Value":string)  [unwired: 2 in, 1 out]
